vi "MDrive_Set_Variable.vi"(3 "error in":errorcluster, 4 "Value":string, 5 "Variable":string, 6 "VISA resource name in":refnum<visa-resource-name>) -> (0 "error out":errorcluster, 1 "number":i32, 2 "VISA resource name out":refnum<visa-resource-name>)   [LabVIEW 2010]
panel:
  out "String":string="\r\n"
  out "substring":string
  out "return count":u32
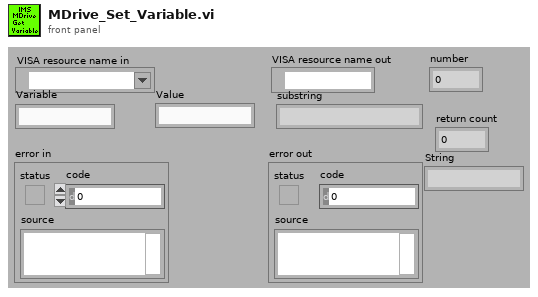
[diagram p1: front panel]
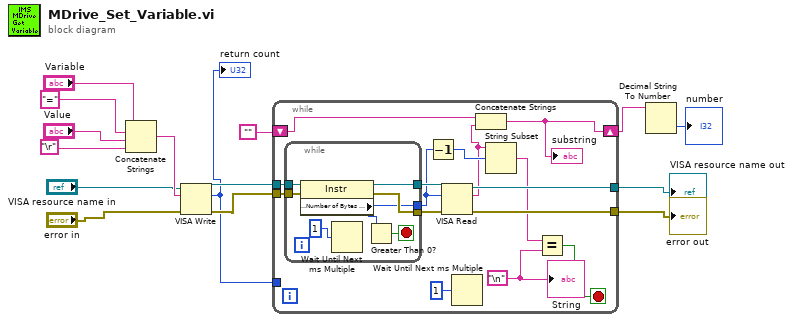
[diagram p0: block diagram]
diagram:
  n1 = Concatenate Strings("Variable", "=" ("string"), "Value", "\r") -> (w15:string)
  n2 = VISA Write(VISA resource name="VISA resource name in", write buffer=w15, error in (no error)="error in") -> (VISA resource name out=w13:refnum<visa-resource-name>, return count=w9:u32, error out=w12:errorcluster)
  "return count" <- w9
  n3 = while {
    tunnel: w13 -> [w28]
    tunnel: w12 -> [w27]
    tunnel: [w26] -> w11
    tunnel: [w25] -> w10
    tunnel: w9 -> [_]
    shift-right: [w17] -> w7
    shift-left: "" -> [w19]
    stop <- w20 stop-if-true
    w16 = "\n"
    n4 = while {
      tunnel: [w37] -> w30
      tunnel: [w36] -> w29
      tunnel: w28 -> [w35]
      tunnel: w27 -> [w34]
      tunnel: [w33] -> w23
      stop <- w32 stop-if-true
      n5 = property class="Instr"(reference=w35, error in=w34) -> (reference out=w37:refnum<visa-resource-name>, error out=w36:errorcluster, "Serial Settings:Number of Bytes at Serial Port"=w33:u32)
      n6 = Wait Until Next ms Multiple(millisecond multiple=u32 1) -> ()  [unwired: 1 out]
      n7 = Greater Than 0?(x=w33) -> (x > 0?=w32:bool)
    }
    n8 = Decrement(x=w23) -> (x-1=w22:u32)
    n9 = VISA Read(VISA resource name=w30, byte count=w23, error in (no error)=w29) -> (VISA resource name out=w26:refnum<visa-resource-name>, read buffer=w18:string, error out=w25:errorcluster)  [unwired: 1 out]
    n10 = Wait Until Next ms Multiple(millisecond multiple=u32 1) -> ()  [unwired: 1 out]
    n11 = Concatenate Strings(w19, w18) -> (w17:string)
    "substring" <- w17
    n12 = String Subset(string=w18, offset (0)=w22) -> (substring=w21:string)  [unwired: 1 in]
    n13 = Equal?(x=w21, y=w16) -> (x = y?=w20:bool)
    "String" <- w16
  }
  "error out" <- w10
  "VISA resource name out" <- w11
  n14 = Decimal String To Number(string=w7) -> (number=→"number":i32)  [unwired: 2 in, 1 out]
